vi "Measure_Buttons.vi"(8 "error in (no error)":errorcluster, 10 "Parameters":string, 11 "reference in":refnum<class "Test_Flux_Capacitor.lvclass">) -> (0 "error out":errorcluster, 2 "Result":bool, 3 "reference out":refnum<class "Test_Flux_Capacitor.lvclass">)   [LabVIEW 2022 SP3, in "Test_Flux_Capacitor.lvlib" / "Test_Flux_Capacitor.lvclass"]
uses:
  Test_Flux_Capacitor.lvclass
  ParameterTypes/Button.ctl
  Components/SwitchBase.lvlibp/SwitchBase.lvclass
  <vilib>/JDP Science/JSONtext/JSONtext.lvlib
panel:
  in  "Parameter_Type":T1
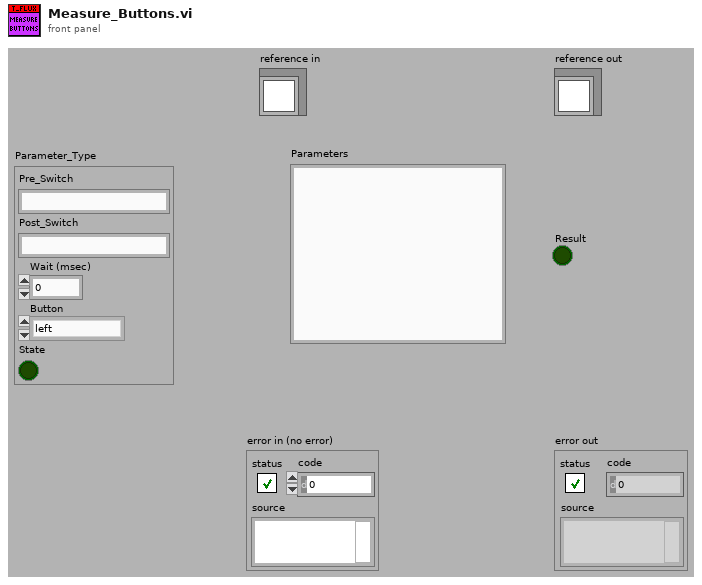
[diagram p1: front panel]
types:
  T1 = typedef "Test_Flux_Capacitor.lvlib/Test_Flux_Capacitor.lvclass/Button.ctl" = cluster{"Pre_Switch":string, "Post_Switch":string, "Wait (msec)":u32, "Button":enum16{"left", "right", "up", "down", "enter", "start"}, "State":bool}
  T2 = typedef "Test_Flux_Capacitor.lvlib/Test_Flux_Capacitor.lvclass/ObjectAttributes.ctl" = cluster{"Config":T3, "DMM":refnum<class "DMM_Keysight_34980A.lvclass">, "LCR":refnum<class "LCR_BK891.lvclass">, "PSU":refnum<class "PSU_Base.lvclass">, "Switch_Manager":refnum<class "SwitchBase.lvclass">, "FRAM":string, "Flux_Capacitor":refnum<class "Flux_Capacitor.lvclass">, "Frequency_Counter":refnum<class "Frequency_Counter_Base.lvclass">, "JTAG":refnum<class "JTAG_Base.lvclass">}
  T3 = typedef "Test_Flux_Capacitor.lvlib/Test_Flux_Capacitor.lvclass/Config.ctl" = cluster{"default":string}
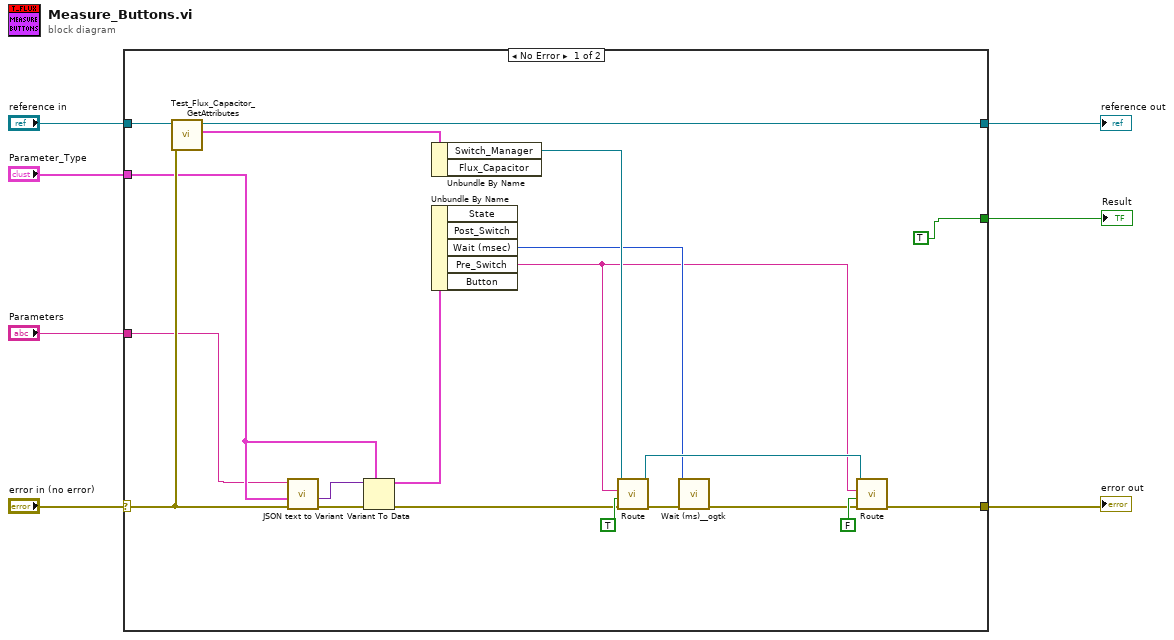
[diagram p0: block diagram]
diagram:
  n1 = case shown="No Error" "error in (no error)" {
    selector: "error in (no error)" -> [w19 w29]
    tunnel: [w9 w29] -> w6
    tunnel: [w26 w28] -> w4
    tunnel: "reference in" -> [w27 w28]
    tunnel: "Parameters" -> [w16 _]
    tunnel: "Parameter_Type" -> [w17 _]
    tunnel: [TRUE _] -> w1
    frame No Error {
      n2 = call "Test_Flux_Capacitor_GetAttributes.vi"("error in (no error)"=w19, "reference in"=w27) -> ("Data"=w25:T2, "reference out"=w26:refnum<class "Test_Flux_Capacitor.lvclass">)  [unwired: 6 in, 2 out]
      n3 = call <vilib>:"JSON text to Variant.vi"("error in (no error)"=w19, "Data Type"=w17, "JSON"=w16) -> ("error out"=w18:errorcluster, "Variant out"=w15:variant)  [unwired: 7 in]
      n4 = Variant To Data(error in=w18, type=w17, Variant=w15) -> (data=w24:T1, error out=w11:errorcluster)
      n5 = Unbundle By Name(w25) -> ("Switch_Manager"=w23:refnum<class "SwitchBase.lvclass">)  [unwired: 1 out]
      n6 = Unbundle By Name(w24) -> ("Wait (msec)"=w21:u32, "Pre_Switch"=w14:string)  [unwired: 3 out]
      n7 = call-dynamic "Route.vi"("error in (no error)"=w11, "Connect"=TRUE, "channel 1"=w14, "reference in"=w23) -> ("error out"=w20:errorcluster, "reference in"=w22:refnum<class "SwitchBase.lvclass">)  [unwired: 6 in]
      n8 = call <userlib>:"Wait (ms)__ogtk.vi"("error in (no error)"=w20, "milliseconds to wait"=w21) -> ("error out"=w10:errorcluster)  [unwired: 8 in, 1 out]
      n9 = call-dynamic "Route.vi"("error in (no error)"=w10, "Connect"=FALSE, "channel 1"=w14, "reference in"=w22) -> ("error out"=w9:errorcluster)  [unwired: 6 in, 1 out]
    }
    frame Error {
    }
  }
  "Result" <- w1
  "error out" <- w6
  "reference out" <- w4
